vi "TestData_Record2Text.vi"(7 "SN":string, 9 "TestTime":dbl, 10 "Result":enum16{"PASS", "FAIL", "INT.", "TOUT"}(ring)=enum."FAIL", 11 "TestRecord":T1={"name_pf"="Product_name", "name_name_ean13"="input SN", "supplier_code"="", "date"="", "time"="", "operater_code"="0", "sw_code"="", "sw_ver"="V10", "test_type"="EOL", "spare"="", "jig_code"="T001", "total_qty"="0", "field_code"="", "test_time"="NA", "test_result"="NA", "serial_number"="input SN", "TestItem"=[]}) -> (2 "Record_Text":string, 3 "OK?":bool=TRUE)   [LabVIEW 2012, in "Lib_UEL.ATE.lvlib" / "Lib_TestData.lvlib"]
uses:
  Lib_TestData.lvlib
panel:
  # "功能说明:\n转换Record簇(结构体)到表格字符串, 以'#'分隔, 并添加Hash到最后以列.\n\n版本信息\nV1.0.0 初始版本."
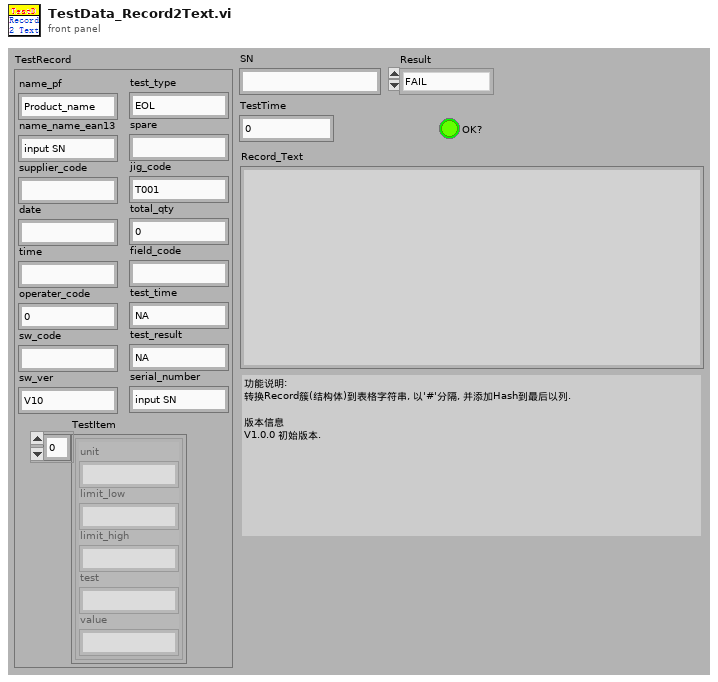
[diagram p1: front panel]
types:
  T1 = cluster{"name_pf":string, "name_name_ean13":string, "supplier_code":string, "date":string, "time":string, "operater_code":string, "sw_code":string, "sw_ver":string, "test_type":string, "spare":string, "jig_code":string, "total_qty":string, "field_code":string, "test_time":string, "test_result":string, "serial_number":string, "TestItem":cluster{"unit":string, "limit_low":string, "limit_high":string, "test":string, "value":string}[]}
  T2 = cluster{"unit":string, "limit_low":string, "limit_high":string, "test":string, "value":string}[]
  T3 = cluster{"unit":string, "limit_low":string, "limit_high":string, "test":string, "value":string}
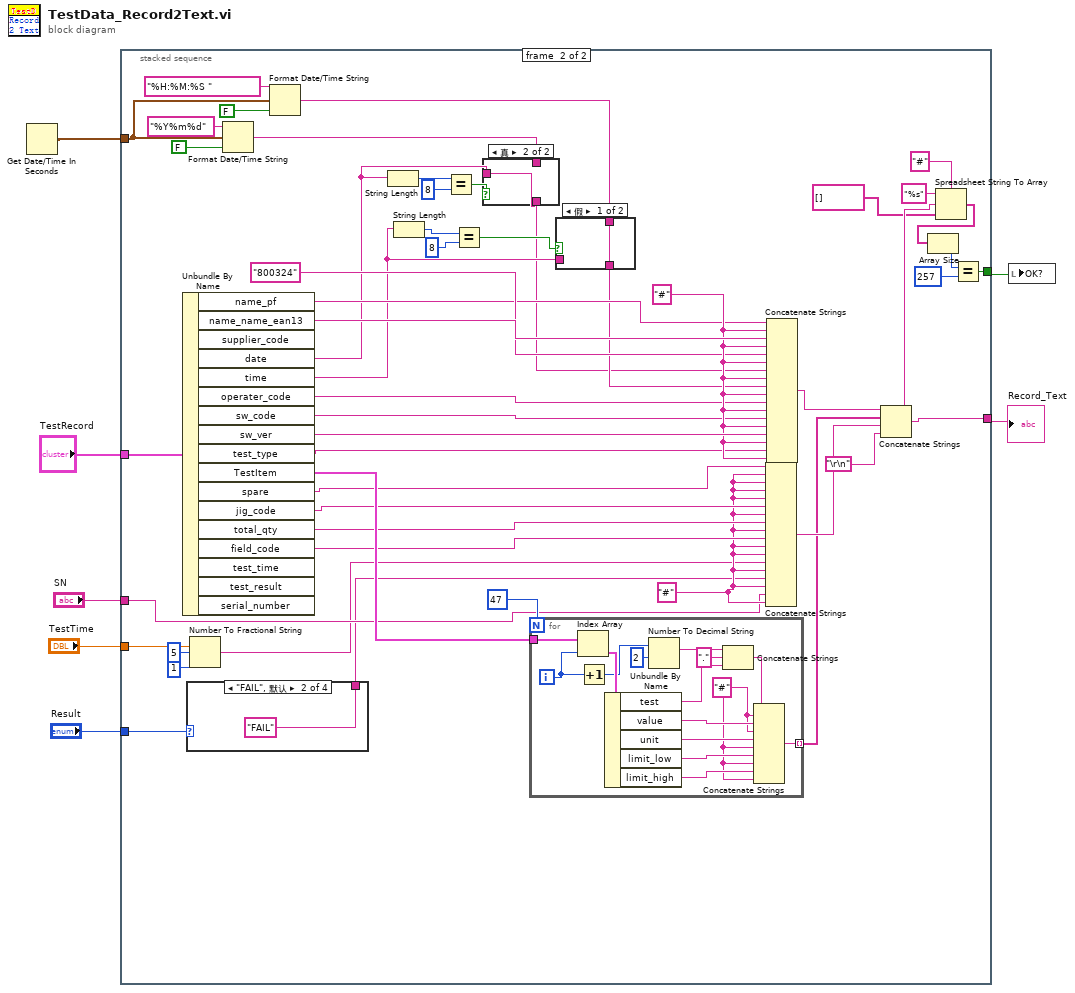
[diagram p0: block diagram]
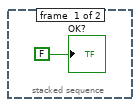
[diagram p2: hidden frame]
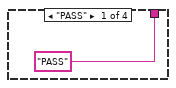
[diagram p3: hidden frame]
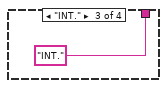
[diagram p4: hidden frame]
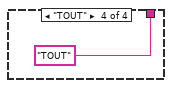
[diagram p5: hidden frame]
diagram:
  n1 = Get Date/Time In Seconds() -> (seconds since 1Jan1904=w7:timestamp)
  n2 = stacked-sequence {
    tunnel: w7 -> [_ w28]
    tunnel: "TestRecord" -> [_ w56]
    tunnel: "Result" -> [_ w38]
    tunnel: "TestTime" -> [_ w37]
    tunnel: "SN" -> [_ w16]
    tunnel: [_ w27] -> w2
    tunnel: [_ w20] -> w1
    frame #0 {
      "OK?" <- FALSE ("OK?")
    }
    frame #1 {
      w29 = "#" ("字符串")
      w51 = "#" ("字符串")
      n3 = Unbundle By Name(w56) -> ("name_pf"=w19:string, "name_name_ean13"=w53:string, "date"=w11:string, "time"=w13:string, "operater_code"=w39:string, "sw_code"=w18:string, "sw_ver"=w52:string, "test_type"=w17:string, "TestItem"=w54:T2, "spare"=w30:string, "jig_code"=w33:string, "total_qty"=w50:string, "field_code"=w49:string)  [unwired: 4 out]
      n4 = case shown="\"FAIL\", 默认" w38 {
        tunnel: ["PASS" ("字符串") "FAIL" ("字符串") "INT." ("字符串") "TOUT" ("字符串")] -> w14
        frame "PASS" {
        }
        frame "FAIL", Default {
        }
        frame "INT." {
        }
        frame "TOUT" {
        }
      }
      n5 = Number To Fractional String(number=w37, width (-)=i16 5 ("宽度(-)"), precision (6)=i16 1 ("精度(6)")) -> (F-format string=w15:string)  [unwired: 1 in]
      n6 = Format Date/Time String(time format string (%c)="%Y%m%d" ("时间格式化字符串(%c)"), seconds (now)=w28, UTC format=FALSE ("UTC格式")) -> (date/time string=w31:string)
      n7 = Format Date/Time String(time format string (%c)="%H:%M:%S " ("时间格式化字符串(%c)"), seconds (now)=w28, UTC format=FALSE ("UTC格式")) -> (date/time string=w32:string)
      n8 = String Length(string=w11) -> (length=w45:i32)
      n9 = String Length(string=w13) -> (length=w42:i32)
      n10 = Equal?(x=w45, y=8) -> (x = y?=w43:bool)
      n11 = Equal?(x=w42, y=8) -> (x = y?=w40:bool)
      n12 = case shown="真" w43 {
        tunnel: [w67 w68] -> w10
        tunnel: w31 -> [w67 _]
        tunnel: w11 -> [_ w68]
        frame False {
        }
        frame True {
        }
      }
      n13 = for {
        N: 47 -> [_]
        tunnel: w54 -> [w83]
        tunnel: [w77] -> w46 mode=indexing
        i -> [w73]
        w75 = "#" ("字符串")
        n14 = Index Array(array=w83, index=w73) -> (element=w82:T3)
        n15 = Increment(x=w73) -> (x+1=w72:i32)
        n16 = Unbundle By Name(w82) -> ("test"=w71:string, "value"=w81:string, "unit"=w80:string, "limit_low"=w79:string, "limit_high"=w78:string)
        n17 = Number To Decimal String(number=w72, width (-)=i16 2 ("宽度(-)")) -> (decimal integer string=w74:string)
        n18 = Concatenate Strings(w74, "." ("字符串"), w71) -> (w69:string)
        n19 = Concatenate Strings(w69, w75, w81, w75, w80, w75, w79, w75, w78, w75) -> (w77:string)
      }
      n20 = case shown="假" w40 {
        tunnel: [w65 w66] -> w12
        tunnel: w32 -> [w65 _]
        tunnel: w13 -> [_ w66]
        frame False {
        }
        frame True {
        }
      }
      n21 = Concatenate Strings(w30, w29, w29, w29, w29, w33, w29, w50, w29, w49, w29, w29, w15, w29, w14, w29, w16, w29) -> (w47:string)
      n22 = Concatenate Strings(w19, w51, w53, w51, "800324" ("字符串"), w51, w10, w51, w12, w51, w39, w51, w18, w51, w52, w51, w17, w51) -> (w48:string)
      n23 = Concatenate Strings(w48, w46, w47, "\r\n") -> (w27:string)
      n24 = Spreadsheet String To Array(delimiter (Tab)="#" ("分隔符(Tab)"), format string="%s" ("格式字符串"), spreadsheet string=w27, array type (2D Dbl)=string[] []) -> (array=w23:string[])
      n25 = Array Size(array=w23) -> (size(s)=w22:i32)
      n26 = Equal?(x=w22, y=257) -> (x = y?=w20:bool)
    }
  }
  "Record_Text" <- w2
  n27 = local write "OK?"(w1) -> ()
